vi "Vision_Left_R10.vi"() -> ()   [LabVIEW 2015]
uses:
  <vilib>/vision/Pattern Matching.llb/IMAQ Curve Parameters.ctl
  <vilib>/vision/Pattern Matching.llb/IMAQ Match Range Setting.ctl
panel:
  out "Avg Scale":dbl=89.2016387939453
  out "Avg Score":dbl=997.8182983398438
  out "Current Search Settings":T3={"Curve Parameters"={"Extraction Mode"=1, "Edge Threshold"=150, "Edge Filter Size"=0, "Min Length"=25, "Row Search Step Size"=15, "Col Search Step Size"=15, "Max Endpoint Gap"=2, "Closed"=TRUE, "Subpixel"=TRUE}, "Match Mode"={"Rotation"=TRUE, "Scale"=TRUE, "Occlusion"=TRUE, "Reserved"=FALSE, "Reserved"=FALSE, "Reserved"=FALSE}, "Range Settings"=[{"Match Constraints"=0, "Min"=-5.0, "Max"=5.0}, {"Match Constraints"=1, "Min"=84.2016387939453, "Max"=94.2016387939453}, {"Match Constraints"=2, "Min"=0.0, "Max"=0.0}], "Number of Matches"=1, "Minimum Match Score"=897.8183, "SubPixel Accuracy"=TRUE, "Adv. Geometric Match Options 2"=[{"Setup Data Item"=20, "Item Value"=0.0}, {"Setup Data Item"=22, "Item Value"=1.0}]} {"Curve Parameters"."Extraction Mode" items=["Normal", "Uniform Regions"]; "Curve Parameters"."Edge Filter Size" items=["Fine", "Normal", "Contour Tracing"]; "Curve Parameters"."Max Endpoint Gap" min=0; "Curve Parameters"."Col Search Step Size" min=1 max=255 step=1; "Curve Parameters"."Row Search Step Size" min=1 max=255 step=1; "Curve Parameters"."Min Length" min=0; "Curve Parameters"."Edge Threshold" min=1 max=350 step=1; "Range Settings"."Max" format="%.2f"; "Range Settings"."Min" format="%.2f"; "Range Settings"."Match Constraints" items=["Rotation Angle (degrees)", "Scale Factor (%)", "Occlusion (%)"]}
  out "Valid Scale History":dbl[](array[numeric])=[89.23128509521484, 89.22906494140625, 89.23128509521484, 89.17756652832031, 89.13899230957031, 89.34435272216797, 89.28369903564453, 89.25519561767578, 89.21601104736328, 89.19574737548828, 89.13480377197266, 89.12804412841797, 89.276611328125, 89.38147735595703, 89.14649200439453, 89.13899230957031, 89.13480377197266, 89.22276306152344, 89.14115142822266, 89.13899230957031] format="%#_13g"
  out "Valid Score History":dbl[](array[numeric])=[997.8182983398438, 997.6611328125, 997.8182983398438, 997.8182983398438, 997.9754638671875, 997.2081298828125, 997.2081298828125, 997.365234375, 997.365234375, 997.8182983398438, 998.1326293945312, 997.6795654296875, 997.365234375, 996.7366333007812, 997.8182983398438, 997.9754638671875, 998.1326293945312, 997.8367309570312, 997.6795654296875, 997.9754638671875] format="%#_13g"
  out "Valid Beacon History - in":bool[](array[boolean])=[TRUE, TRUE, TRUE, TRUE, TRUE, TRUE, TRUE, TRUE, TRUE, TRUE, TRUE, TRUE, TRUE, TRUE, TRUE, TRUE, TRUE, TRUE, TRUE, TRUE]
  out "Startup Flag":bool
  out "Current Tempalte State":enum16{"Short Range", "Long Range"}(ring)
  out "Lock Status":bool=TRUE
  out "Y Coordinates":sgl[](array[numeric])=[0.0, 150.09842, 152.7592, 152.49298, 0.0]
  out "X Coordinates":sgl[](array[numeric])=[0.0, 96.87595, 158.4174, 215.82172, 0.0]
  out "Beacons Found":bool[](array[boolean])=[FALSE, TRUE, TRUE, TRUE, FALSE]
  out "Left Image out":T4(plugin-control)
  in  "Initial State":enum16{"Short Range", "Long Range"}(ring)
  in  "History Size":i32=20
  in  "INITIAL Search Settings":T3={"Curve Parameters"={"Extraction Mode"=1, "Edge Threshold"=150, "Edge Filter Size"=0, "Min Length"=25, "Row Search Step Size"=15, "Col Search Step Size"=15, "Max Endpoint Gap"=2, "Closed"=TRUE, "Subpixel"=TRUE}, "Match Mode"={"Rotation"=TRUE, "Scale"=TRUE, "Occlusion"=TRUE, "Reserved"=FALSE, "Reserved"=FALSE, "Reserved"=FALSE}, "Range Settings"=[{"Match Constraints"=0, "Min"=-5.0, "Max"=5.0}, {"Match Constraints"=1, "Min"=50.0, "Max"=150.0}, {"Match Constraints"=2, "Min"=0.0, "Max"=25.0}], "Number of Matches"=1, "Minimum Match Score"=750.0, "SubPixel Accuracy"=TRUE, "Adv. Geometric Match Options 2"=[{"Setup Data Item"=20, "Item Value"=0.0}, {"Setup Data Item"=22, "Item Value"=1.0}]} {"Curve Parameters"."Extraction Mode" items=["Normal", "Uniform Regions"]; "Curve Parameters"."Edge Filter Size" items=["Fine", "Normal", "Contour Tracing"]; "Curve Parameters"."Max Endpoint Gap" min=0; "Curve Parameters"."Col Search Step Size" min=1 max=255 step=1; "Curve Parameters"."Row Search Step Size" min=1 max=255 step=1; "Curve Parameters"."Min Length" min=0; "Curve Parameters"."Edge Threshold" min=1 max=350 step=1; "Range Settings"."Max" format="%.2f"; "Range Settings"."Min" format="%.2f"; "Range Settings"."Match Constraints" items=["Rotation Angle (degrees)", "Scale Factor (%)", "Occlusion (%)"]; "Adv. Geometric Match Options 2"."Setup Data Item" items=["Curve Extraction Mode", "Curve Edge Threshold", "Curve Edge Filter Size", "Min Curve Length", "Curve Row Search Step Size", "Curve Col Search Step Size", "Curve Max Endpoint Gap", "Extract Closed Curves", "Enable Subpixel Curve Extraction", "Enable Correlation Score", "Enable Subpixel Accuracy", "Subpixel Iterations", "Subpixel Tolerance", "Initial Match List Length", "Enable Target Template Curve Score", "Min Match Separation Distance", "Min Match Separation Angle", "Min Match Separation Scale", "Max Match Overlap", "Enable Coarse Result", "Enable Calibration Support", "Enable Contrast Reversal", "Search Strategy", "Refinement Match Factor", "Subpixel Match Factor"]}
  # "Range"
  # "Range"
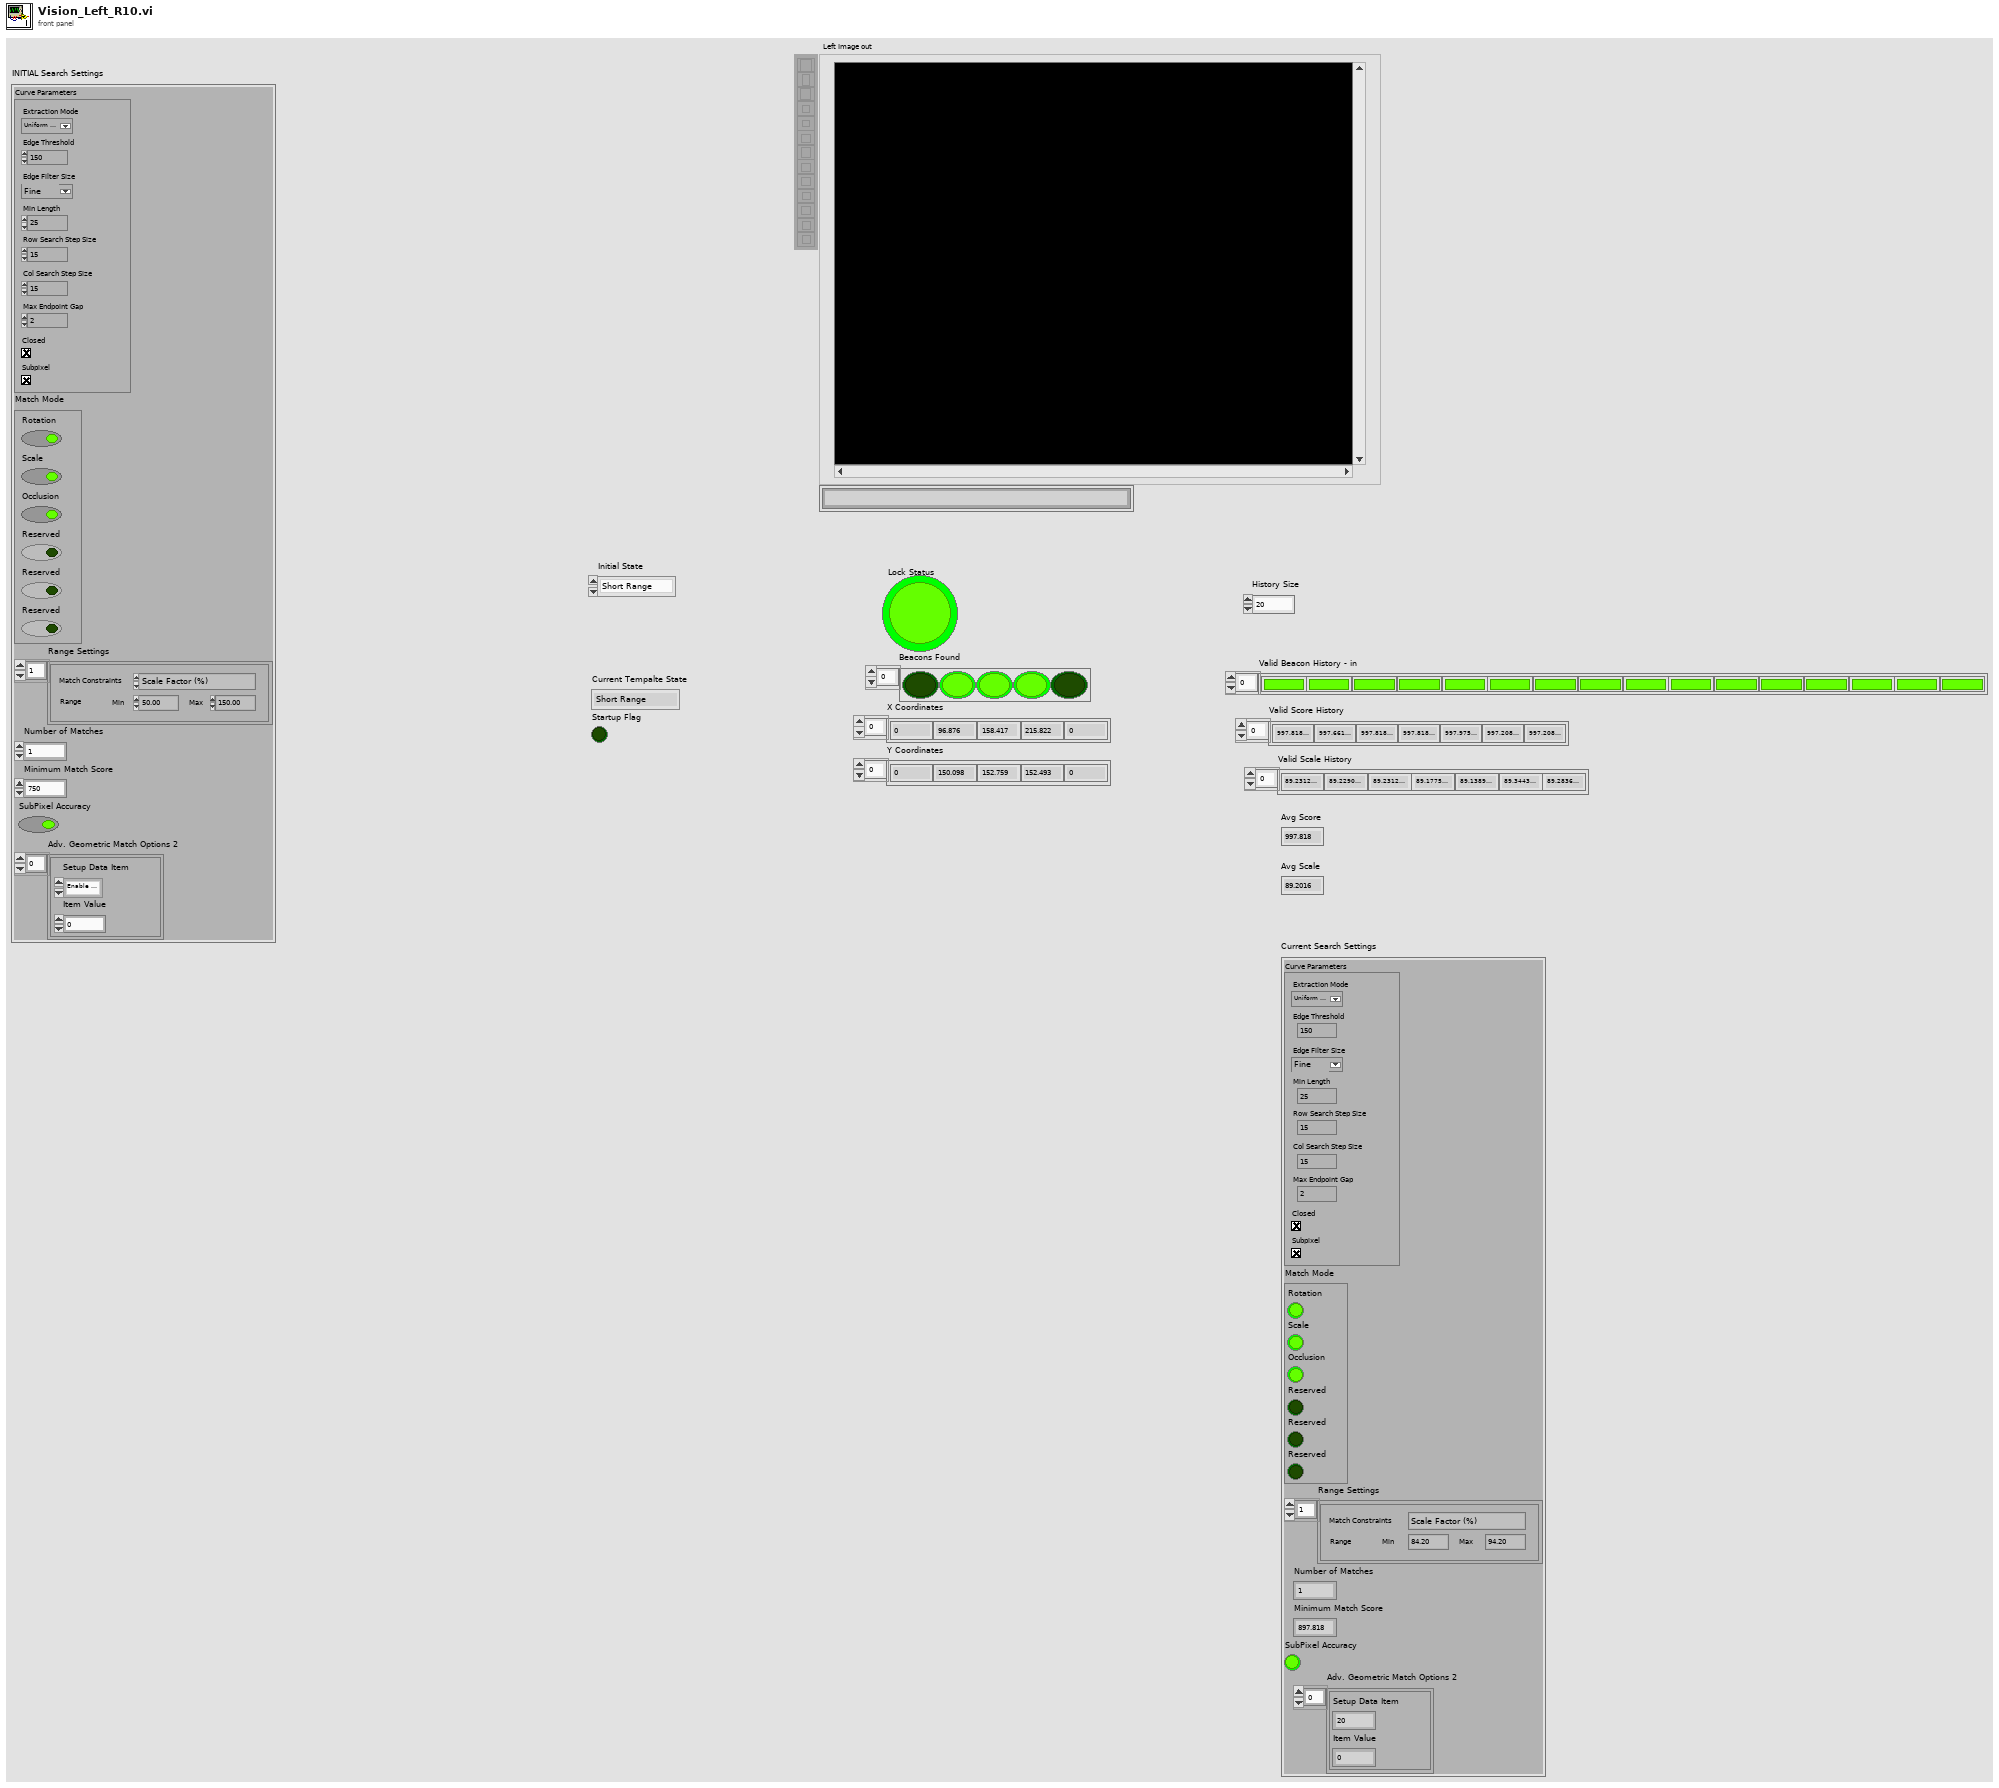
[diagram p1: front panel]
types:
  T1 = typedef "IMAQ Curve Parameters.ctl" = cluster{"Extraction Mode":u32, "Edge Threshold":i32, "Edge Filter Size":u32, "Min Length":i32, "Row Search Step Size":i32, "Col Search Step Size":i32, "Max Endpoint Gap":i32, "Closed":bool, "Subpixel":bool}
  T2 = typedef "IMAQ Match Range Setting.ctl" = cluster{"Match Constraints":u32, "Min":dbl, "Max":dbl}
  T3 = cluster{"Curve Parameters":T1, "Match Mode":cluster{"Rotation":bool, "Scale":bool, "Occlusion":bool, "Reserved":bool, "Reserved":bool, "Reserved":bool}, "Range Settings":T2[], "Number of Matches":i32, "Minimum Match Score":sgl, "SubPixel Accuracy":bool, "Adv. Geometric Match Options 2":cluster{"Setup Data Item":u16, "Item Value":dbl}[]}
  T4 = typedef "IMAQ Image.ctl" = refnum<image>
  T5 = typedef "Image Type" = u32
  T6 = typedef "ROI Descriptor" = cluster{"Global Rectangle":i32[], "Contours":cluster{"ID":enum32{"External", "Internal"}, "Type":u32, "Coordinates":i32[]}[]}
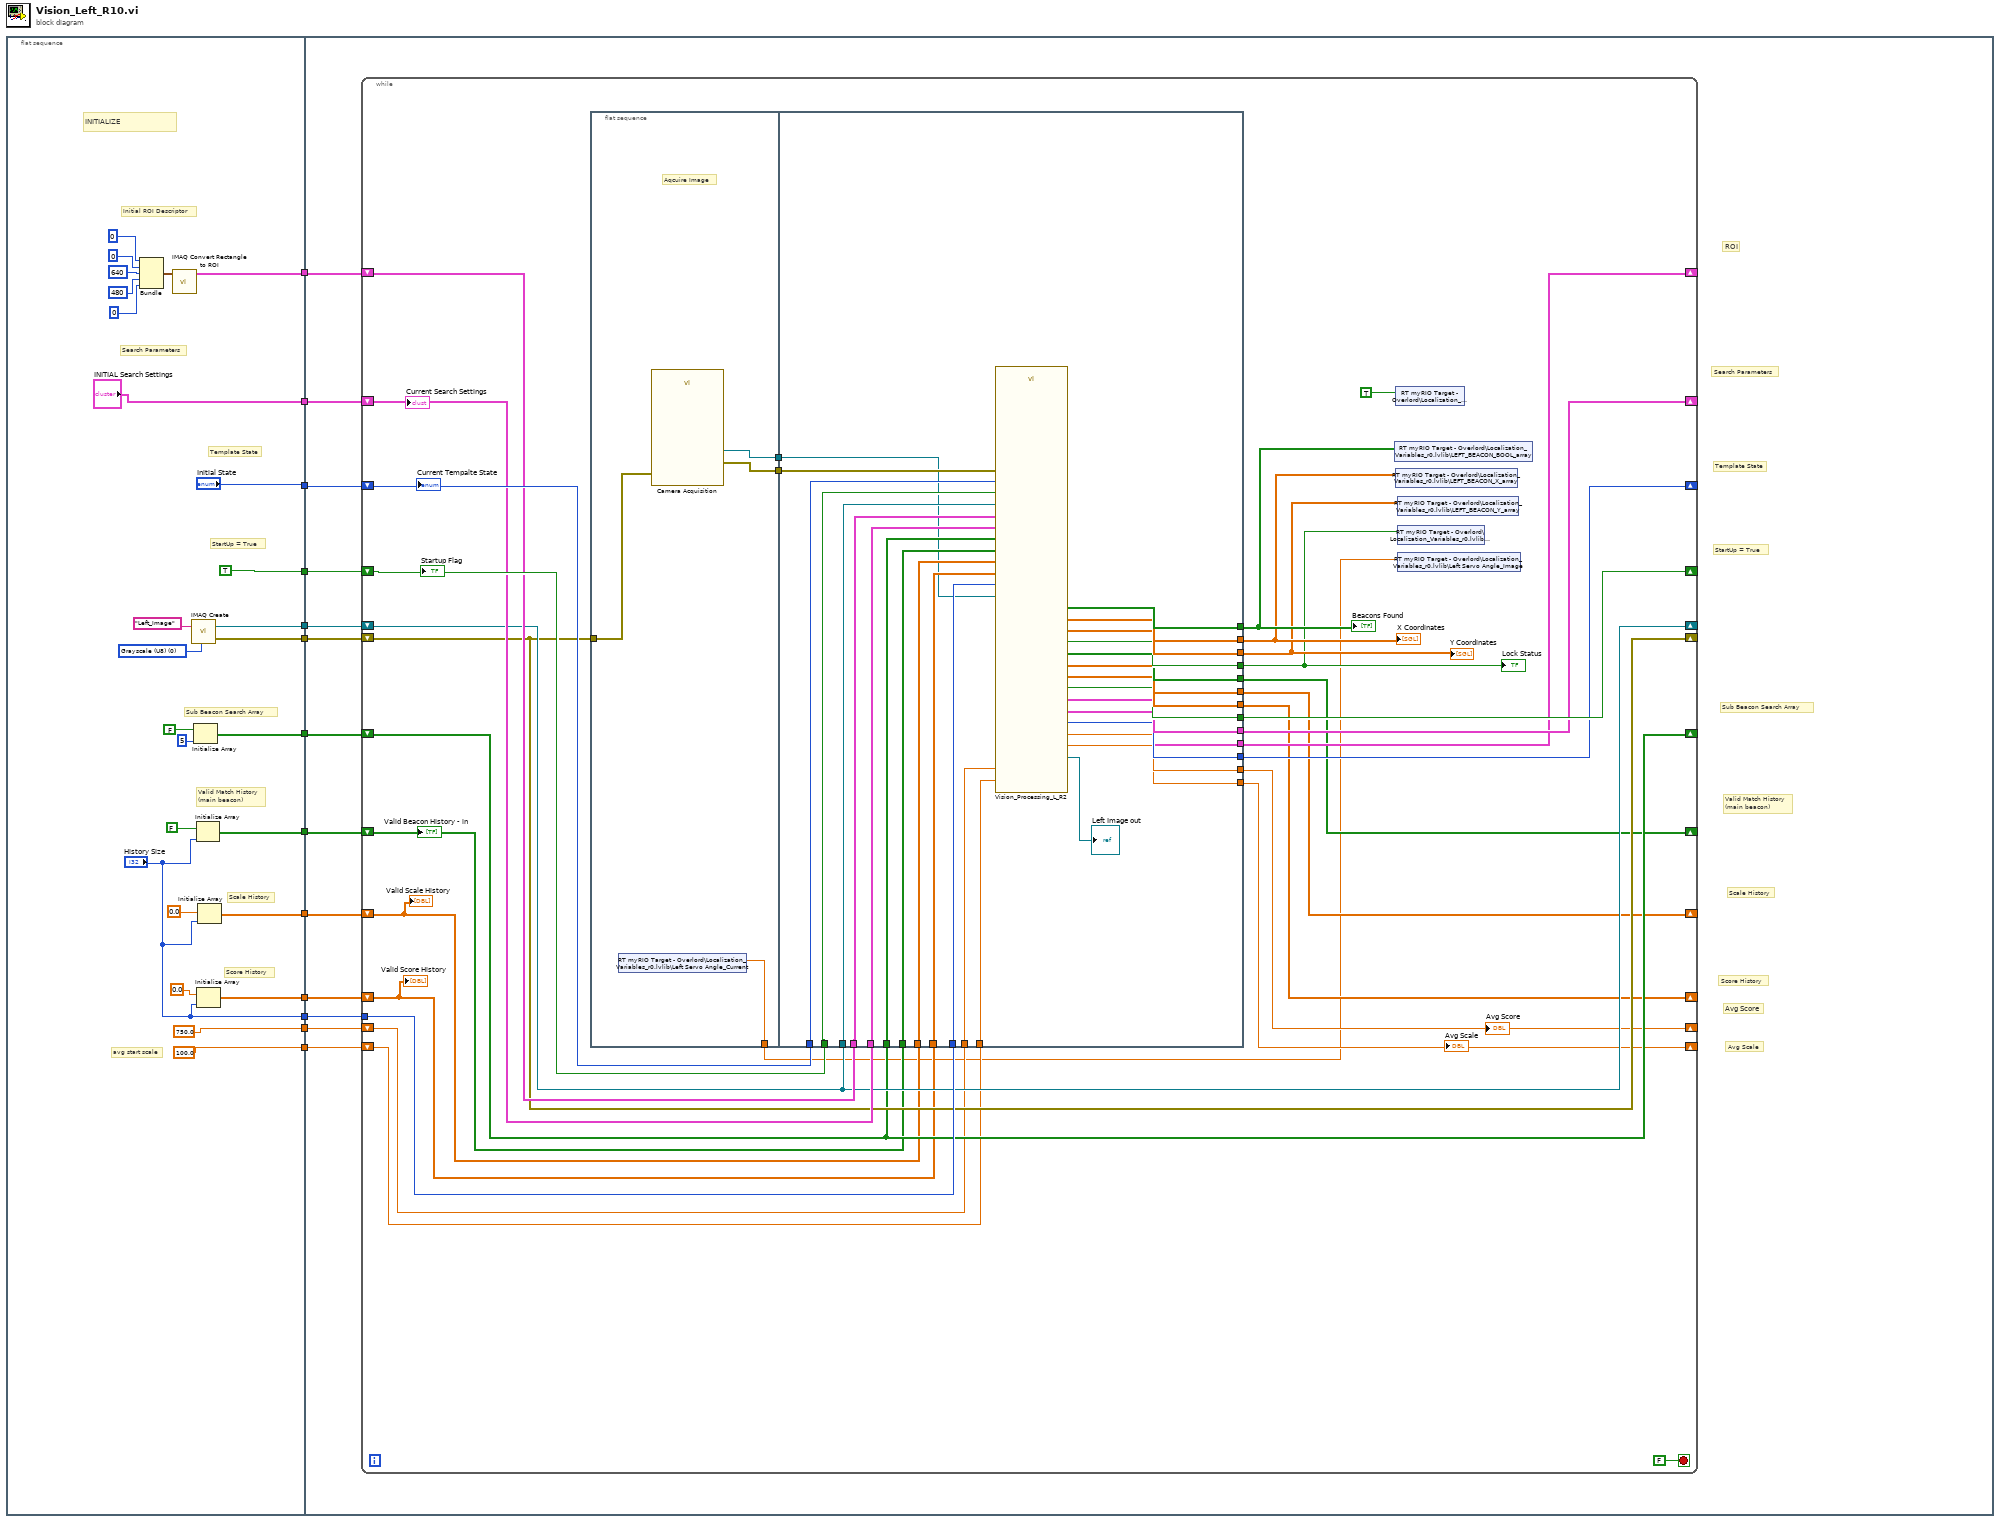
[diagram p0: block diagram]
diagram:
  n1 = flat-sequence {
    tunnel: [w26] -> w13
    tunnel: ["INITIAL Search Settings"] -> w12
    tunnel: ["Initial State"] -> w11
    tunnel: [TRUE] -> w10
    tunnel: [w23] -> w9
    tunnel: [w22] -> w8
    tunnel: [w21] -> w7
    tunnel: [w20] -> w6
    tunnel: [w19] -> w5
    tunnel: [w18] -> w4
    tunnel: ["History Size"] -> w3
    tunnel: [750.0] -> w2
    tunnel: [100.0] -> w1
    tunnel: w13 -> [w52]
    tunnel: w12 -> [w51]
    tunnel: w11 -> [w50]
    tunnel: w10 -> [w49]
    tunnel: w9 -> [w44]
    tunnel: w8 -> [w43]
    tunnel: w7 -> [w48]
    tunnel: w6 -> [w47]
    tunnel: w5 -> [w46]
    tunnel: w4 -> [w45]
    tunnel: w3 -> [w42]
    tunnel: w2 -> [w41]
    tunnel: w1 -> [w40]
    frame #0 {
      w33 = T5 0 items=["Grayscale (U8)", "Grayscale (I16)", "Grayscale (SGL)", "Complex (CSG)", "RGB (U32)", "HSL (U32)", "RGB (U64)", "Grayscale (U16)"] ("Image Type")
      # "avg start scale"
      # "Score History"
      # "Scale History"
      # "Valid Match History\n(main beacon)"
      # "Sub Beacon Search Array"
      # "Template State"
      # "Search Parameters"
      # "StartUp = True"
      # "Initial ROI Descriptor"
      # "INITIALIZE"
      n2 = Bundle(0, 0, 640, 480, 0) -> (w32:cluster{i32, i32, i32, i32, i32})  [unwired: 1 in]
      n3 = call "IMAQ Convert Rectangle to ROI"("Rectangle"=w32) -> ("ROI Descriptor"=w26:T6)  [unwired: 8 in, 1 out]
      n4 = call "IMAQ Create"("Image Name"="Left_Image", "Image Type"=w33) -> ("New Image"=w23:T4, "error out"=w22:errorcluster)  [unwired: 3 in]
      n5 = Initialize Array(FALSE, 5 ("dimension size")) -> (w21:bool[])
      n6 = Initialize Array(FALSE, "History Size") -> (w20:bool[])
      n7 = Initialize Array(0.0, "History Size") -> (w18:dbl[])
      n8 = Initialize Array(0.0, "History Size") -> (w19:dbl[])
    }
    frame #1 {
      # "Avg Scale"
      # "Avg Score"
      # "Score History"
      # "Scale History"
      # "Valid Match History\n(main beacon)"
      # "Sub Beacon Search Array"
      # "StartUp = True"
      # "Template State"
      # "Search Parameters"
      # "ROI"
      n9 = while {
        shift-right: [w70] -> _
        shift-left: w52 -> [w78]
        shift-right: [w71] -> _
        shift-left: w51 -> [w77]
        shift-right: [w72] -> _
        shift-left: w50 -> [w81]
        shift-right: [w73] -> _
        shift-left: w49 -> [w79]
        shift-right: [w69] -> _
        shift-left: w48 -> [w69]
        shift-right: [w68] -> _
        shift-left: w47 -> [w65]
        shift-right: [w67] -> _
        shift-left: w46 -> [w64]
        shift-right: [w66] -> _
        shift-left: w45 -> [w63]
        shift-right: [w75] -> _
        shift-left: w44 -> [w75]
        shift-right: [w74] -> _
        shift-left: w43 -> [w74]
        tunnel: w42 -> [w76]
        shift-right: [w62] -> _
        shift-left: w41 -> [w60]
        shift-right: [w61] -> _
        shift-left: w40 -> [w59]
        stop <- FALSE stop-if-true
        n10 = flat-sequence {
          tunnel: w74 -> [w87]
          tunnel: [w86] -> w82
          tunnel: [w85] -> w80
          tunnel: [w84] -> w54
          tunnel: w82 -> [w92]
          tunnel: w81 -> [w114]
          tunnel: w80 -> [w115]
          tunnel: w79 -> [w113]
          tunnel: w75 -> [w112]
          tunnel: w78 -> [w111]
          tunnel: w77 -> [w110]
          tunnel: w69 -> [w109]
          tunnel: w65 -> [w108]
          tunnel: w64 -> [w107]
          tunnel: w63 -> [w106]
          tunnel: w76 -> [w105]
          tunnel: w60 -> [w89]
          tunnel: [w103] -> w58
          tunnel: [w102] -> w57
          tunnel: [w101] -> w56
          tunnel: [w100] -> w55
          tunnel: [w99] -> w68
          tunnel: [w98] -> w67
          tunnel: [w97] -> w66
          tunnel: [w96] -> w73
          tunnel: [w95] -> w71
          tunnel: [w93] -> w70
          tunnel: [w94] -> w72
          tunnel: [w91] -> w62
          tunnel: [w90] -> w61
          tunnel: w59 -> [w88]
          frame #0 {
            # "Aqcuire Image"
            n11 = shared-variable "RT myRIO Target - Overlord\\Localization_Variables_r0.lvlib\\Left Servo Angle_Current"() -> (w84:dbl)  [unwired: 1 in, 1 out]
            n12 = call "Camera Acquisition"("error in"=w87) -> ("Image Out"=w86:T4, "error out"=w85:errorcluster)  [unwired: 24 in, 1 out]
          }
          frame #1 {
            n13 = call "Vision_Processing_L_R2.vi"("Current State"=w114, "Image Dst"=w112, "Inpute Image"=w92, "Startup Flag"=w113, "Valid Beacon History - in"=w108, "Current ROI Descriptor"=w111, "Avg Score - Last"=w89, "error in (no error)"=w115, "Current Settings"=w110, "Sub Beacon Search Enable"=w109, "Avg Scale - Last"=w88, "Valid Score History"=w106, "Valid Scale History"=w107, "History Size"=w105) -> ("Valid Scale History\nOut"=w98:dbl[], "Avg Scale"=w90:dbl, "Avg Score"=w91:dbl, "Valid Score History\nOut"=w97:dbl[], "Valid Beacon History\nOut"=w99:bool[], "Y Coordinates"=w101:sgl[], "Beacons Found"=w103:bool[], "X Coordinates"=w102:sgl[], "Next Main ROI Descriptor"=w93:T6, "Lock Status"=w100:bool, "Startup Flag - out"=w96:bool, "New Settings"=w95:T3, "Next State"=w94:enum16{"Short Range", "Long Range"}, "Right Image 2"=→"Left Image out":T4)
          }
        }
        n14 = shared-variable "RT myRIO Target - Overlord\\Localization_Variables_r0.lvlib\\LEFT_BEACON_BOOL_array"(w58) -> ()  [unwired: 1 in, 1 out]
        n15 = shared-variable "RT myRIO Target - Overlord\\Localization_Variables_r0.lvlib\\Left_Flag"(TRUE) -> ()  [unwired: 1 in, 1 out]
        n16 = shared-variable "RT myRIO Target - Overlord\\Localization_Variables_r0.lvlib\\LEFT_BEACON_X_array"(w57) -> ()  [unwired: 1 in, 1 out]
        n17 = shared-variable "RT myRIO Target - Overlord\\Localization_Variables_r0.lvlib\\LEFT_BEACON_Y_array"(w56) -> ()  [unwired: 1 in, 1 out]
        n18 = shared-variable "RT myRIO Target - Overlord\\Localization_Variables_r0.lvlib\\Image Lock - L"(w55) -> ()  [unwired: 1 in, 1 out]
        n19 = shared-variable "RT myRIO Target - Overlord\\Localization_Variables_r0.lvlib\\Left Servo Angle_Image"(w54) -> ()  [unwired: 1 in, 1 out]
        "Beacons Found" <- w58
        "X Coordinates" <- w57
        "Y Coordinates" <- w56
        "Lock Status" <- w55
        "Current Tempalte State" <- w81
        "Startup Flag" <- w79
        "Valid Scale History" <- w64
        "Valid Beacon History - in" <- w65
        "Valid Score History" <- w63
        "Current Search Settings" <- w77
        "Avg Score" <- w62
        "Avg Scale" <- w61
      }
    }
  }
